vi "Prepare Stack.vi"(8 "error in (no error)":errorcluster, 10 "Stack Info":T1, 11 "TIFF in":refnum<class "TIFF.lvclass">) -> (0 "error out":errorcluster, 3 "TIFF out":refnum<class "TIFF.lvclass">)   [LabVIEW 2018, in "BinaryTIFF.lvlib" / "TIFF.lvclass"]
uses:
  TIFF.lvclass
  TIFF.lvclass/TIFF.ctl
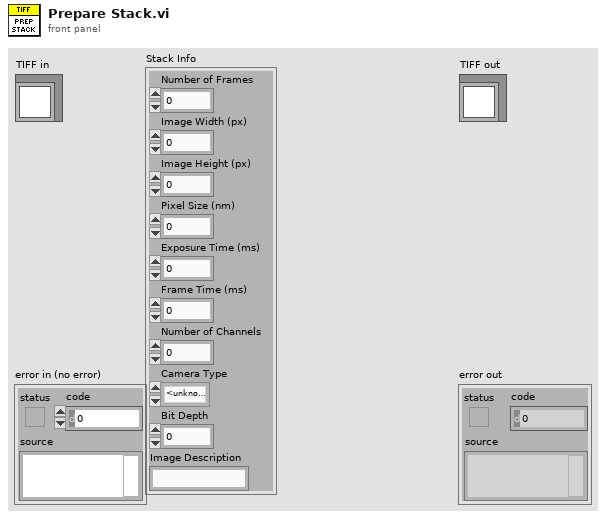
[diagram p1: front panel]
types:
  T1 = cluster{"Number of Frames":u32, "Image Width (px)":u32, "Image Height (px)":u32, "Pixel Size (nm)":dbl, "Exposure Time (ms)":dbl, "Frame Time (ms)":dbl, "Number of Channels":u32, "Camera Type":enum16{"<unknown>", "Evolve 512", "Orca-Flash 4.0 V2"}, "Bit Depth":u32, "Image Description":string}
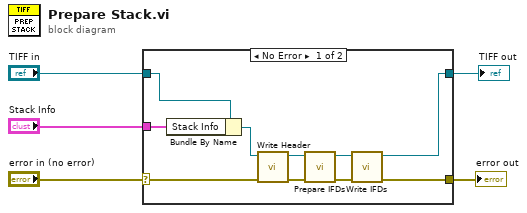
[diagram p0: block diagram]
diagram:
  n1 = case shown="No Error" "error in (no error)" {
    selector: "error in (no error)" -> [w13 w17]
    tunnel: [w6 w17] -> w4
    tunnel: [w7 w16] -> w2
    tunnel: "TIFF in" -> [w15 w16]
    tunnel: "Stack Info" -> [w8 _]
    frame No Error {
      n2 = Bundle By Name(cluster=w15, "Stack Info"=w8) -> (w14:refnum<class "TIFF.lvclass">)
      n3 = call-dynamic "Write Header.vi"("error in (no error)"=w13, "TIFF in"=w14) -> ("error out"=w11:errorcluster, "TIFF out"=w12:refnum<class "TIFF.lvclass">)  [unwired: 8 in]
      n4 = call-dynamic "Prepare IFDs.vi"("error in (no error)"=w11, "TIFF in"=w12) -> ("error out"=w9:errorcluster, "TIFF out"=w10:refnum<class "TIFF.lvclass">)  [unwired: 8 in]
      n5 = call-dynamic "Write IFDs.vi"("error in (no error)"=w9, "TIFF in"=w10) -> ("error out"=w6:errorcluster, "TIFF out"=w7:refnum<class "TIFF.lvclass">)  [unwired: 8 in]
    }
    frame Error {
    }
  }
  "error out" <- w4
  "TIFF out" <- w2
